vi "Test ID pulse.vi"(10 "MUX RELAY":refnum<visa-resource-name>="COM3", 11 "DSO1072B":refnum<visa-resource-name>="USB0::0x0957::0x0588::CN55040431::INSTR") -> (2 "PWIDTH":dbl format="%#_6f", 3 "MAX AMP":dbl format="%#_6f")   [LabVIEW 2011]
panel:
  out "PWIDTH":string
  out "MAX AMP":string
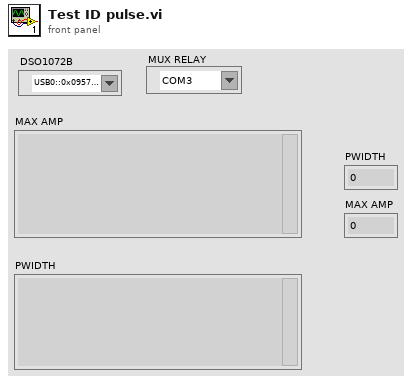
[diagram p1: front panel]
types:
  T1 = enum32{"Set Relay", "Append Relay", "Clear Relay", "Manual Cmd"}
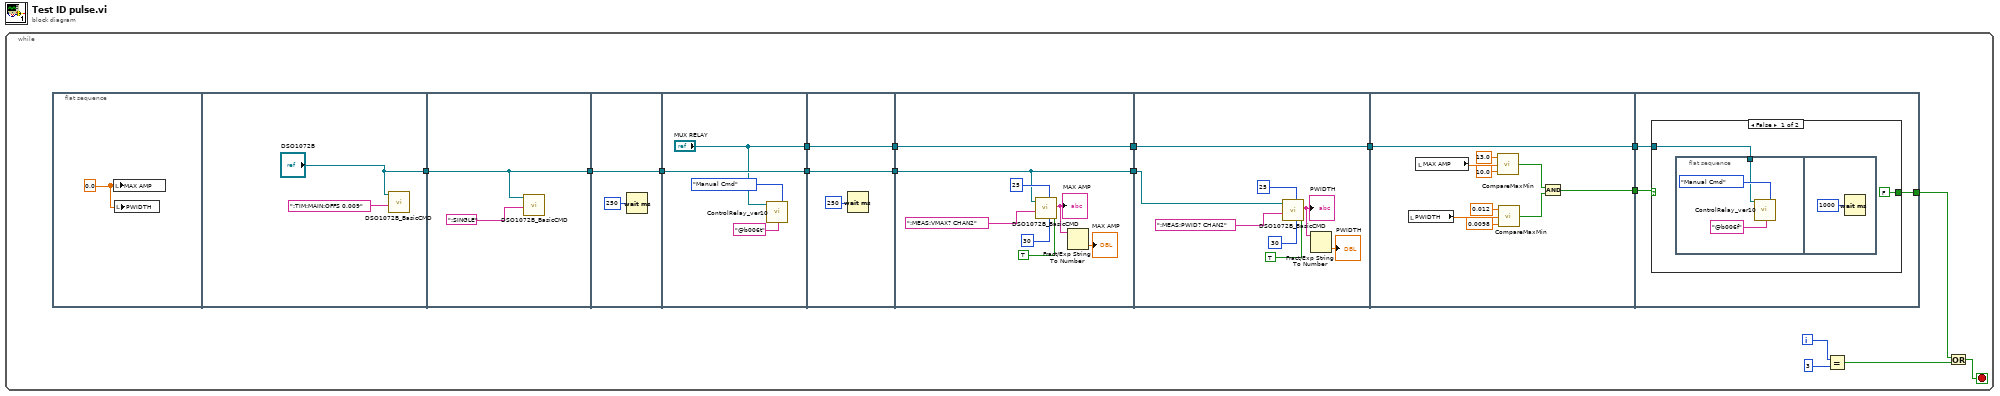
[diagram p0: block diagram]
diagram:
  n1 = while {
    i -> [w5]
    stop <- w3 stop-if-true
    n2 = flat-sequence {
      tunnel: ["DSO1072B"] -> w17
      tunnel: [w21] -> w16
      tunnel: w17 -> [w21]
      tunnel: [w23] -> w15
      tunnel: w16 -> [w23]
      tunnel: w15 -> [w28]
      tunnel: [w28] -> w14
      tunnel: ["MUX RELAY"] -> w13
      tunnel: w14 -> [w31]
      tunnel: [w31] -> w12
      tunnel: [w29] -> w11
      tunnel: w13 -> [w29]
      tunnel: w12 -> [w34]
      tunnel: [w35] -> w10
      tunnel: w11 -> [w35]
      tunnel: [w34] -> w9
      tunnel: w10 -> [w47]
      tunnel: [w47] -> w8
      tunnel: w9 -> [w42]
      tunnel: w8 -> [w57]
      tunnel: [w57] -> w7
      tunnel: [w48] -> w6
      tunnel: w7 -> [w60]
      tunnel: w6 -> [w59]
      tunnel: [w58] -> w2
      frame #0 {
        w18 = 0.0
        n3 = local write "MAX AMP"(w18) -> ()
        n4 = local write "PWIDTH"(w18) -> ()
      }
      frame #1 {
        n5 = call "DSO1072B_BasicCMD.vi"("DSO1072B CMD"=":TIM:MAIN:OFFS 0.009", "VISA resource name In"="DSO1072B") -> ()  [unwired: 7 in, 3 out]
      }
      frame #2 {
        n6 = call "DSO1072B_BasicCMD.vi"("DSO1072B CMD"=":SINGLE", "VISA resource name In"=w21) -> ()  [unwired: 7 in, 3 out]
      }
      frame #3 {
        n7 = Wait (ms)(milliseconds to wait=u32 250) -> ()  [unwired: 1 out]
      }
      frame #4 {
        n8 = call "ControlRelay_ver10.vi"("VISA session"="MUX RELAY", "write buffer"="@b006t", "Relay Setting"=T1."Manual Cmd") -> ()  [unwired: 13 in, 4 out]
      }
      frame #5 {
        n9 = Wait (ms)(milliseconds to wait=u32 250) -> ()  [unwired: 1 out]
      }
      frame #6 {
        n10 = call "DSO1072B_BasicCMD.vi"("AutoRead"=TRUE, "Delay(mS)"=u32 30, "byte count"=u32 25, "DSO1072B CMD"=":MEAS:VMAX? CHAN2", "VISA resource name In"=w34) -> ("read buffer"=w32:string)  [unwired: 4 in, 2 out]
        "MAX AMP" <- w32
        n11 = Fract/Exp String To Number(string=w32) -> (number=→"MAX AMP":dbl)  [unwired: 3 in, 1 out]
      }
      frame #7 {
        n12 = call "DSO1072B_BasicCMD.vi"("AutoRead"=TRUE, "Delay(mS)"=u32 30, "byte count"=u32 25, "DSO1072B CMD"=":MEAS:PWID? CHAN2", "VISA resource name In"=w42) -> ("read buffer"=w41:string)  [unwired: 4 in, 2 out]
        "PWIDTH" <- w41
        n13 = Fract/Exp String To Number(string=w41) -> (number=→"PWIDTH":dbl)  [unwired: 3 in, 1 out]
      }
      frame #8 {
        n14 = local read "PWIDTH"() -> (w51:dbl)
        n15 = local read "MAX AMP"() -> (w56:dbl)
        n16 = call "CompareMaxMin.vi"("Min"=10.0, "X"=w56, "Max"=13.0) -> ("OutCompare"=w50:bool)
        n17 = call "CompareMaxMin.vi"("Min"=0.0098, "X"=w51, "Max"=0.012) -> ("OutCompare"=w49:bool)
        n18 = And(x=w50, y=w49) -> (x .and. y?=w48:bool)
      }
      frame #9 {
        n19 = case shown="False" w59 {
          selector: w59 -> [_ w67]
          tunnel: w60 -> [w62 _]
          tunnel: [FALSE w67] -> w58
          frame False {
            n20 = flat-sequence {
              tunnel: w62 -> [w63]
              frame #0 {
                n21 = call "ControlRelay_ver10.vi"("VISA session"=w63, "write buffer"="@b006f", "Relay Setting"=T1."Manual Cmd") -> ()  [unwired: 13 in, 4 out]
              }
              frame #1 {
                n22 = Wait (ms)(milliseconds to wait=u32 1000) -> ()  [unwired: 1 out]
              }
            }
          }
          frame True {
          }
        }
      }
    }
    n23 = Equal?(x=w5, y=3) -> (x = y?=w1:bool)
    n24 = Or(x=w2, y=w1) -> (x .or. y?=w3:bool)
  }
